vi "DSF.Engine.Framework.Get Tx Transfer Groups.vi"(11 "Framework in":refnum<class "DSF.Engine.Framework.lvclass">) -> (2 "Tx Transfer Groups":refnum<class "DSF.Engine.Transfer Group.lvclass">[](array[class]), 3 "Framework out":refnum<class "DSF.Engine.Framework.lvclass">)   [LabVIEW 2017]
uses:
  DSF.Engine.Framework.lvclass
  Transfer/DSF.Engine.Transfer Group.lvclass
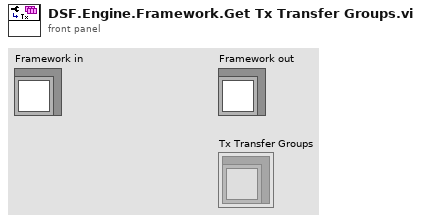
[diagram p1: front panel]
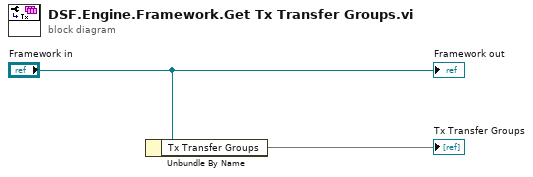
[diagram p0: block diagram]
diagram:
  n1 = Unbundle By Name("Framework in") -> ("Tx Transfer Groups"=→"Tx Transfer Groups")
  "Framework out" <- "Framework in"
